vi "test_aliasing_200MHz.vi"() -> ()   [LabVIEW 2013]
uses:
  <vilib>/measure/maspectr.llb/Power Spectrum and PSD Export Mode.ctl
  <vilib>/measure/maspectr.llb/FFT Power Spectrum and PSD for 1 Chan.vi
  <vilib>/measure/maspectr.llb/FFT Power Spectrum and PSD for 1 Chan (CDB).vi
  <vilib>/measure/NI_MAPro.lvlib
panel:
  out "after filter 2":cluster{"f0":dbl, "df":dbl, "magnitude":dbl[]}(graph)
  out "mixer signal":cluster{"f0":dbl, "df":dbl, "magnitude":dbl[]}(graph)
  out "signal":cluster{"f0":dbl, "df":dbl, "magnitude":dbl[]}(graph)
  out "after mixing":cluster{"f0":dbl, "df":dbl, "magnitude":dbl[]}(graph)
  out "after filter":cluster{"f0":dbl, "df":dbl, "magnitude":dbl[]}(graph)
  out "Array":fxp<+/-,20,16>[](array[numeric])
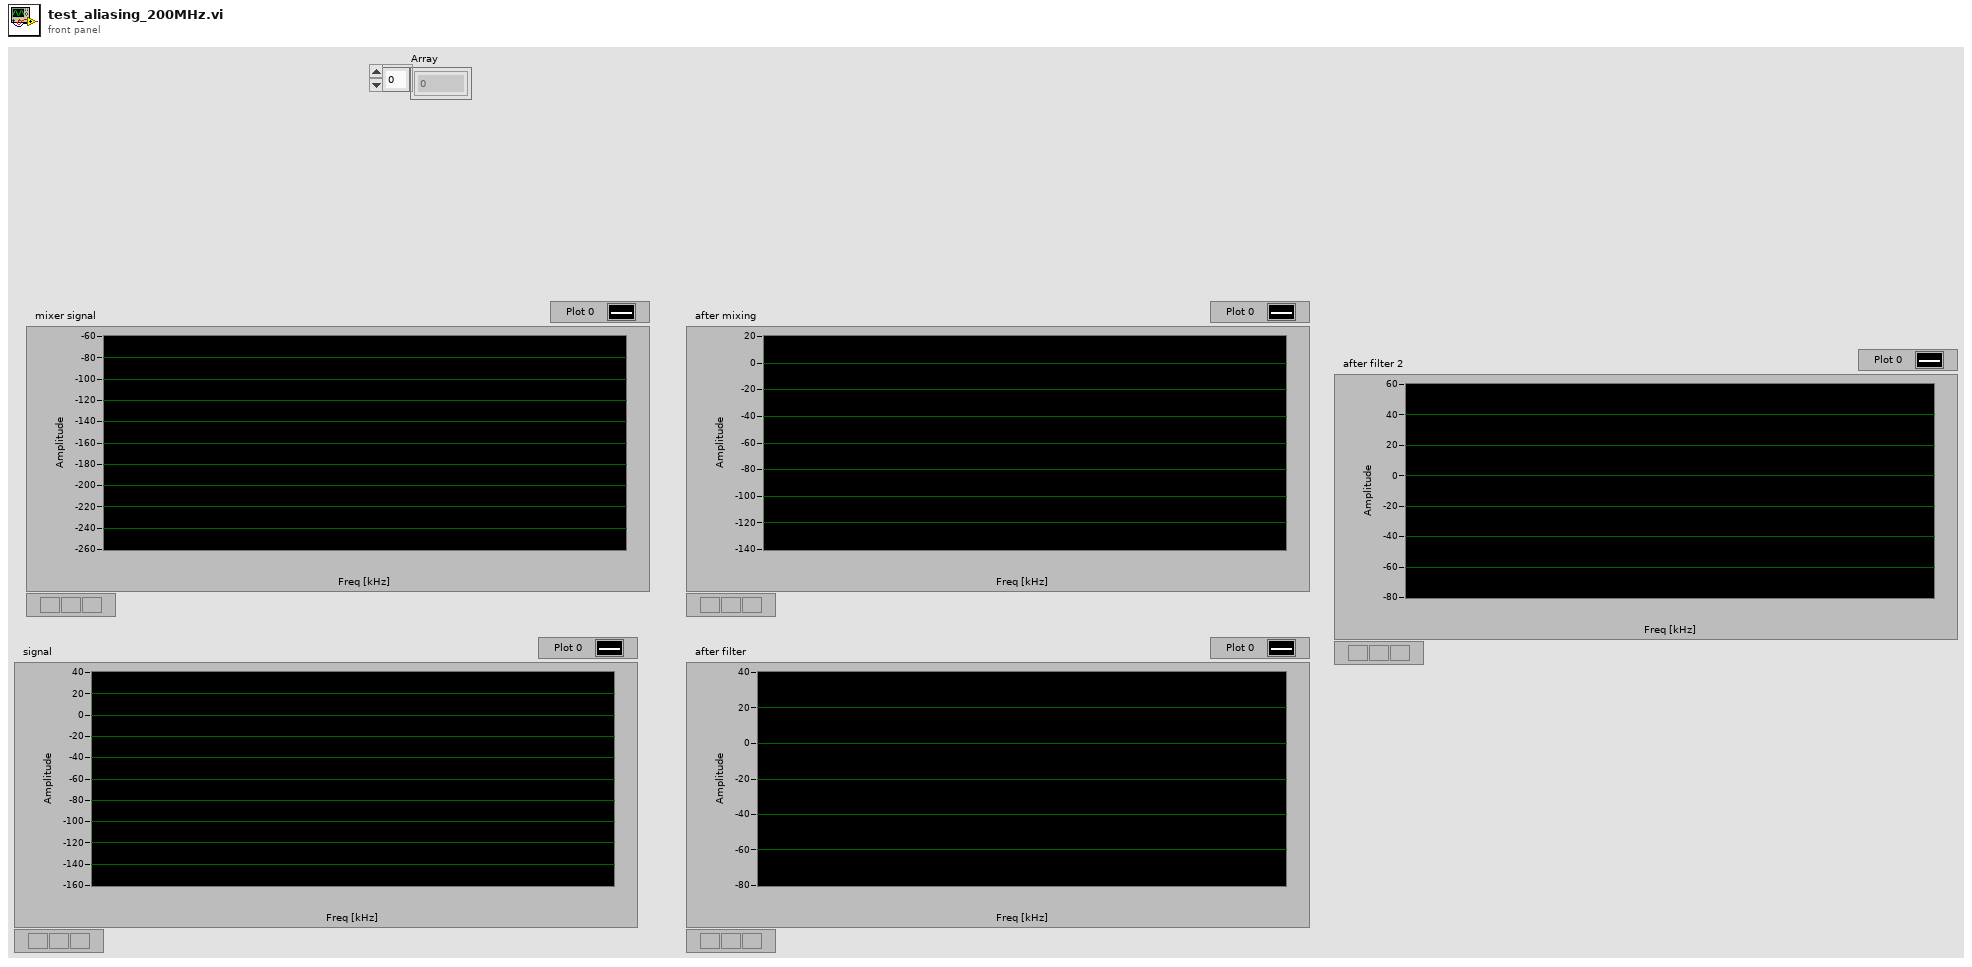
[diagram p1: front panel]
types:
  T1 = typedef "NI_MAPro.lvlib/Power Spectrum and PSD Export Mode.ctl" = u16
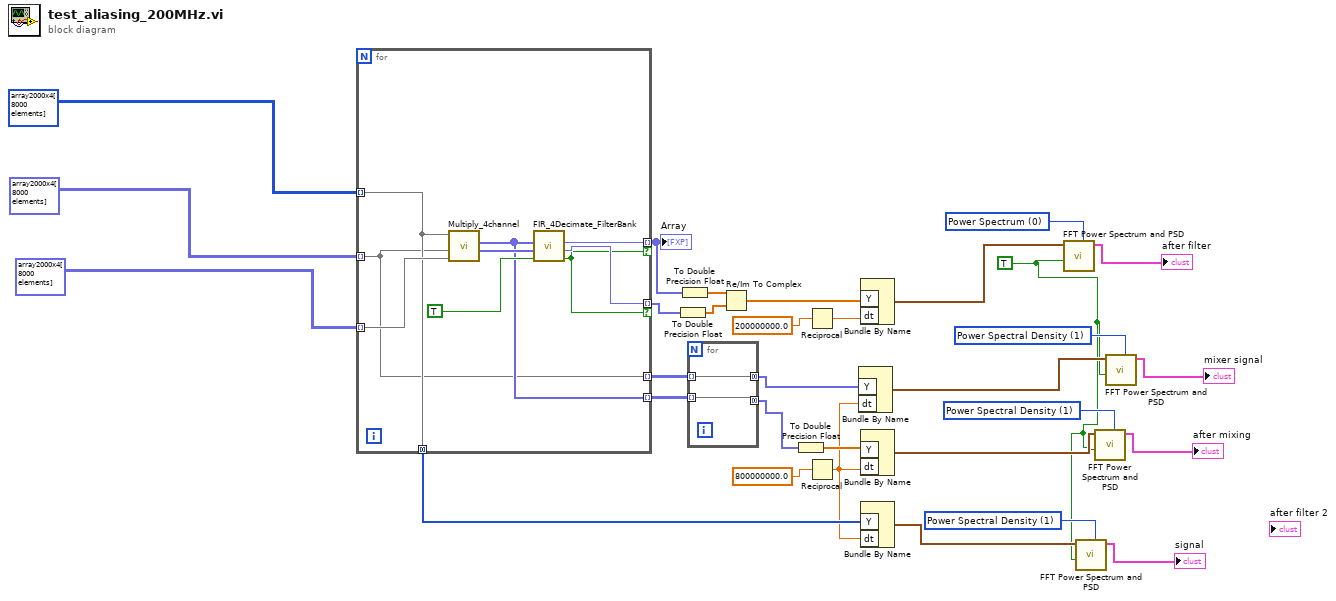
[diagram p0: block diagram]
diagram:
  w10 = TRUE ("dB On (F)")
  w14 = T1 1 items=["Power Spectrum", "Power Spectral Density"] ("export mode")
  w19 = T1 1 items=["Power Spectrum", "Power Spectral Density"] ("export mode")
  w24 = T1 1 items=["Power Spectrum", "Power Spectral Density"] ("export mode")
  w31 = T1 0 items=["Power Spectrum", "Power Spectral Density"] ("export mode")
  n1 = for {
    tunnel: i16[][] array2000x4[8000 elements] ("simulated 2D") -> [w35] mode=indexing
    tunnel: fxp<+/-,16,0>[][] array2000x4[8000 elements] ("Cosine out") -> [w34] mode=indexing
    tunnel: fxp<+/-,16,0>[][] array2000x4[8000 elements] ("Sine out") -> [w38] mode=indexing
    tunnel: [w37] -> w8 mode=indexing if=w32
    tunnel: [w36] -> w22 mode=indexing
    tunnel: [w35] -> w16 mode=concatenating
    tunnel: [w34] -> w15 mode=indexing
    tunnel: [w33] -> w7 mode=indexing if=w32
    n2 = call "Multiply_4channel.vi"("DDS Sine"=w38, "DDS Cosine"=w34, "Signal Input"=w35) -> ("Q output"=w40:fxp<+/-,16,14>[], "I output"=w36:fxp<+/-,16,14>[])  [unwired: 7 in]
    n3 = call "FIR_4Decimate_FilterBank.vi"("data valid in"=TRUE ("valid in"), "Q in"=w40, "I in"=w36) -> ("data valid out"=w32:bool, "Q out"=w33:fxp<+/-,16,14>, "I out"=w37:fxp<+/-,16,14>)  [unwired: 6 in]
  }
  "Array" <- w8
  n4 = To Double Precision Float(number=w7) -> (double precision float=w6:dbl[])
  n5 = To Double Precision Float(number=w8) -> (double precision float=w9:dbl[])
  n6 = for {
    tunnel: w22 -> [w42] mode=indexing
    tunnel: [w42] -> w21 mode=concatenating
    tunnel: w15 -> [w41] mode=indexing
    tunnel: [w41] -> w1 mode=concatenating
  }
  n7 = Re/Im To Complex(1:w6, 2:w9) -> (0:w5:cdb[])
  n8 = To Double Precision Float(number=w21) -> (double precision float=w23:dbl[])
  n9 = Reciprocal(x=200000000.0 ("dt")) -> (1/x=w27:dbl)
  n10 = Reciprocal(x=800000000.0 ("dt")) -> (1/x=w12:dbl)
  n11 = Bundle By Name("Y"=w1, "dt"=w12) -> (w11:waveform(dbl))  [unwired: 1 in]
  n12 = Bundle By Name("Y"=w5, "dt"=w27) -> (w30:waveform(cdb))  [unwired: 1 in]
  n13 = Bundle By Name("Y"=w23, "dt"=w12) -> (w20:waveform(dbl))  [unwired: 1 in]
  n14 = Bundle By Name("Y"=w16, "dt"=w12) -> (w17:waveform(i16))  [unwired: 1 in]
  n15 = call-poly <vilib>:"FFT Power Spectrum and PSD.vi"("export mode"=w31, "dB On (F)"=w10, "time signal"=w30) -> ("Power Spectrum / PSD"=→"after filter":cluster{"f0":dbl, "df":dbl, "magnitude":dbl[]})  [unwired: 5 in, 3 out]
  n16 = call-poly <vilib>:"FFT Power Spectrum and PSD.vi"("export mode"=w19, "dB On (F)"=w10, "time signal"=w17) -> ("Power Spectrum / PSD"=→"signal":cluster{"f0":dbl, "df":dbl, "magnitude":dbl[]})  [unwired: 5 in, 3 out]
  n17 = call-poly <vilib>:"FFT Power Spectrum and PSD.vi"("export mode"=w24, "dB On (F)"=w10, "time signal"=w20) -> ("Power Spectrum / PSD"=→"after mixing":cluster{"f0":dbl, "df":dbl, "magnitude":dbl[]})  [unwired: 5 in, 3 out]
  n18 = call-poly <vilib>:"FFT Power Spectrum and PSD.vi"("export mode"=w14, "dB On (F)"=w10, "time signal"=w11) -> ("Power Spectrum / PSD"=→"mixer signal":cluster{"f0":dbl, "df":dbl, "magnitude":dbl[]})  [unwired: 5 in, 3 out]
